vi "Init.vi"(8 "error in (no error)":errorcluster, 11 "Status_Text_Indicator":refnum<vi>) -> (0 "error out":errorcluster)   [LabVIEW 2020, in "status_text_indicator.lvlib"]
uses:
  Status_Text_Indicator.lvlib
  PTRL/String_Control/string_control.lvlib
panel:
  # "Development\ncontrols/indicators useful for development and testing, but which are not outputs of the VI"
  # "Input\nInputs to the VI"
  # "Output\nOutputs of the VI"
  # "Description\n\nBlank VI with error handling case. \n\nSummarize the use of this VI in this space."
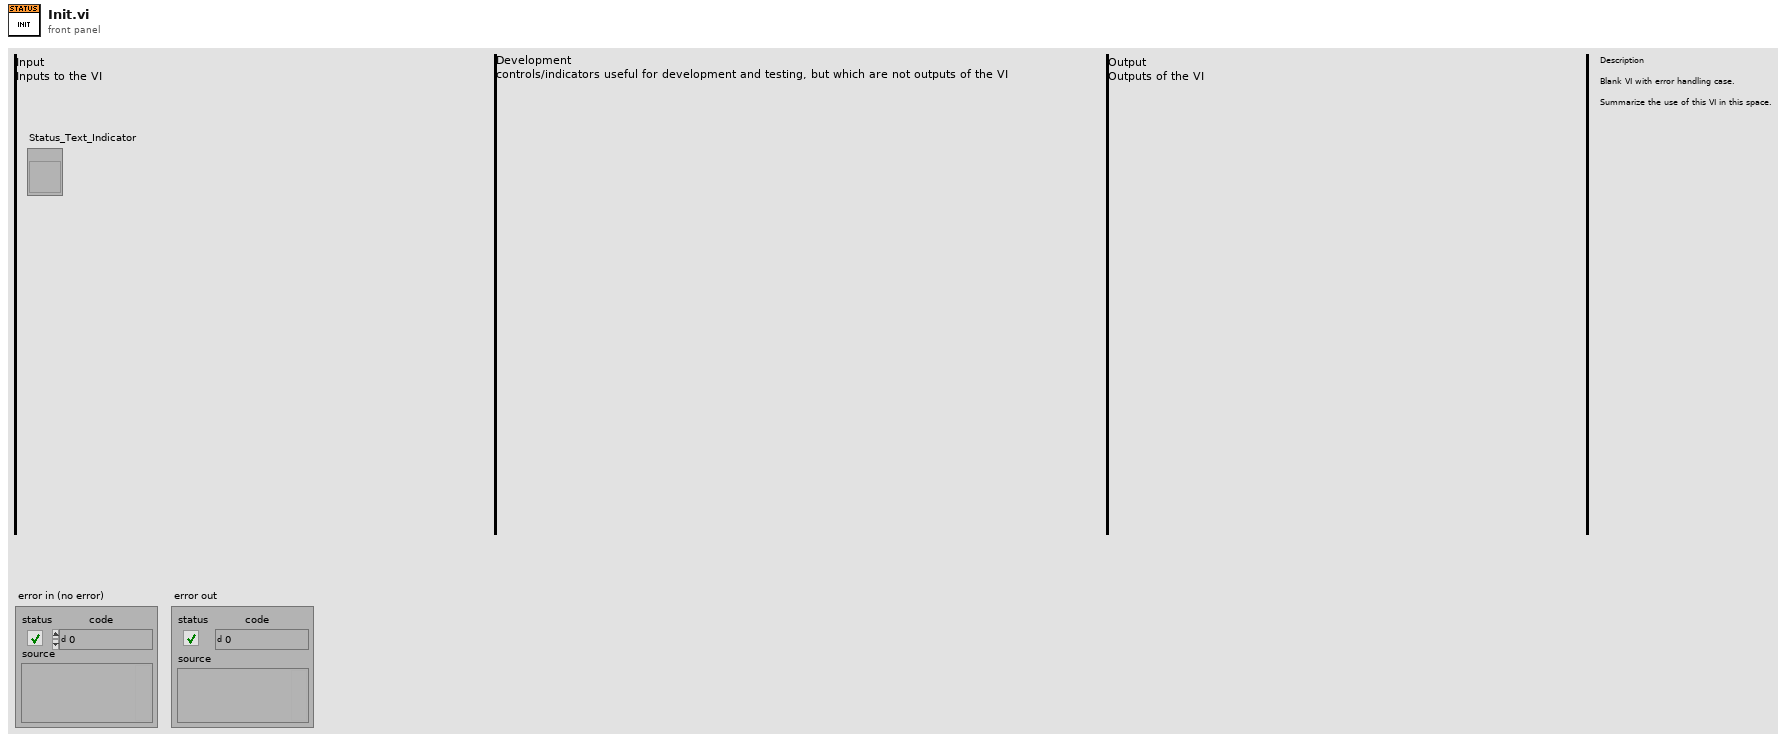
[diagram p1: front panel]
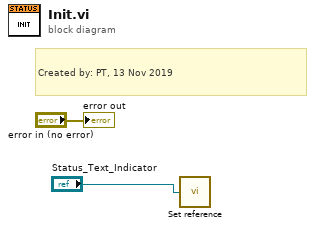
[diagram p0: block diagram]
diagram:
  # "Created by: PT, 13 Nov 2019"
  n1 = call "Set reference.vi"("String_Control"="Status_Text_Indicator") -> ()
  "error out" <- "error in (no error)"
